vi "Initialize MeasurementLink Session.vi"(7 "remote connection options":T2, 8 "error in":errorcluster, 9 "initialize and close session behavior":T1, 10 "session initialization parameters":T3, 11 "instrument in":refnum<class "Session Factory.lvclass">) -> (0 "error out":errorcluster, 2 "session out":variant, 3 "instrument out":refnum<class "Session Factory.lvclass">)   [LabVIEW 2020, in "MeasurementLink niDCPower.lvlib" / "Session Factory.lvclass"]
uses:
  Session Factory.lvclass
  MeasurementLink Instrument/ISession Factory/Session Initialization Parameters.ctl
  MeasurementLink Instrument/ISession Factory/Remote Connection Options.ctl
  MeasurementLink Instrument/ISession Factory/Initialize and Close Session Behavior.ctl
  Session Factory.lvclass/Session Factory.ctl
  MeasurementLink Measurement Server/Helpers/Error Strings Global Internal.vi
  MeasurementLink Instrument/ISession Factory/ISession Factory.lvclass
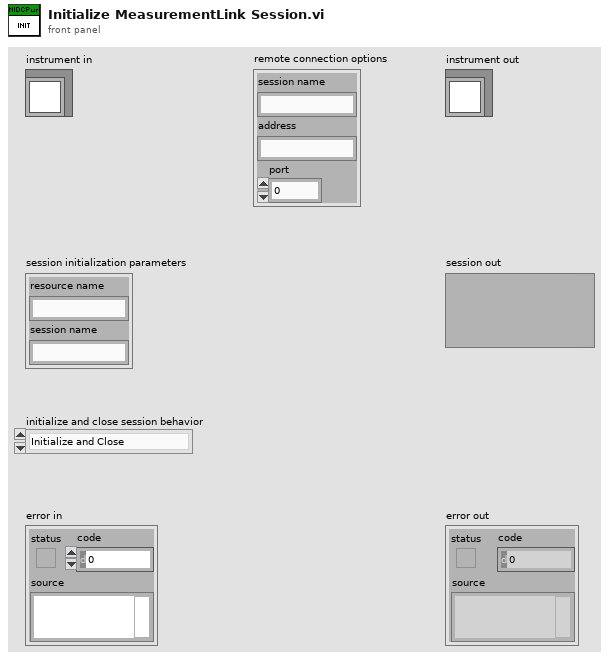
[diagram p1: front panel]
types:
  T1 = typedef "MeasurementLink Instrument.lvlib/ISession Factory.lvclass/Initialize and Close Session Behavior.ctl" = enum16{"Initialize and Close", "Attach and Detach", "Initialize and Detach", "Attach and Close"}
  T2 = typedef "MeasurementLink Instrument.lvlib/ISession Factory.lvclass/Remote Connection Options.ctl" = cluster{"session name":string, "address":string, "port":u32}
  T3 = typedef "MeasurementLink Instrument.lvlib/ISession Factory.lvclass/Session Initialization Parameters.ctl" = cluster{"resource name":string, "session name":string}
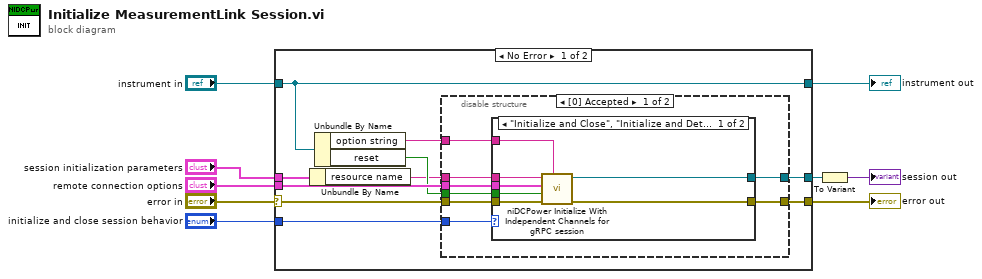
[diagram p0: block diagram]
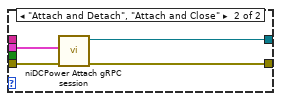
[diagram p2: hidden frame]
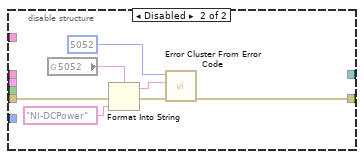
[diagram p3: hidden frame]
diagram:
  n1 = case shown="No Error" "error in" {
    selector: "error in" -> [w16 w46]
    tunnel: [w15 w46] -> w8
    tunnel: "instrument in" -> [w13 w47]
    tunnel: [w13 w47] -> w6
    tunnel: "initialize and close session behavior" -> [w19 _]
    tunnel: "remote connection options" -> [w18 _]
    tunnel: "session initialization parameters" -> [w14 _]
    tunnel: [w17 _] -> w2
    frame No Error {
      n2 = Unbundle By Name(w14) -> ("resource name"=w10:string)
      n3 = Unbundle By Name(w13) -> ("option string"=w12:string, "reset"=w11:bool)
      n4 = disable-structure shown="[0] Accepted" {
        disable-tunnel: w19 -> [w27 _]
        disable-tunnel: w18 -> [w26 _]
        disable-tunnel: [w25 _] -> w17
        disable-tunnel: w16 -> [w24 w40]
        disable-tunnel: [w23 w39] -> w15
        disable-tunnel: w10 -> [w22 _]
        disable-tunnel: w12 -> [w21 _]
        disable-tunnel: w11 -> [w20 _]
        frame Enabled {
          n5 = case shown="\"Initialize and Close\", \"Initialize and Detach\"" w27 {
            tunnel: w26 -> [w33 w38]
            tunnel: [w32 w37] -> w25
            tunnel: w24 -> [w34 w36]
            tunnel: [w31 w35] -> w23
            tunnel: w22 -> [w30 _]
            tunnel: w21 -> [w29 _]
            tunnel: w20 -> [w28 _]
            frame "Initialize and Close", "Initialize and Detach" {
              n6 = call <instrlib>:"niDCPower Initialize With Independent Channels for gRPC session.vi"("option string"=w29, "error in (no error)"=w34, "reset (false)"=w28, "gRPC options"=w33, "resource name"=w30) -> ("error out"=w31:errorcluster, "instrument handle out"=w32:refnum<k15>)  [unwired: 5 in]
            }
            frame "Attach and Detach", "Attach and Close" {
              n7 = call <instrlib>:"niDCPower Attach gRPC session.vi"("error in (no error)"=w36, "gRPC options"=w38) -> ("error out"=w35:errorcluster, "instrument handle out"=w37:refnum<k15>)  [unwired: 8 in]
            }
          }
        }
        frame Disabled {
          n8 = global read "Error Strings Global Internal.vi" "5052"() -> (w44:string)
          n9 = Format Into String(format string=w44, error in=w40, "NI-DCPower") -> (resulting string=w41:string, error out=w42:errorcluster)  [unwired: 1 in]
          n10 = call <vilib>:"Error Cluster From Error Code.vi"("error in (no error)"=w42, "error message (\"\")"=w41, "error code (0)"=5052) -> ("error out"=w39:errorcluster)  [unwired: 6 in]
        }
      }
    }
    frame Error {
    }
  }
  "error out" <- w8
  "instrument out" <- w6
  n11 = To Variant(anything=w2) -> (Variant=→"session out":variant)
